vi "Create Controls within Form.vi"() -> ()   [LabVIEW 2012, in "Form.lvlib"]
uses:
  Form.lvlib
  System.Windows.Forms
panel:
  in  "停止":bool
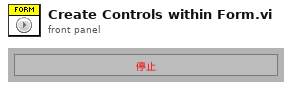
[diagram p1: front panel]
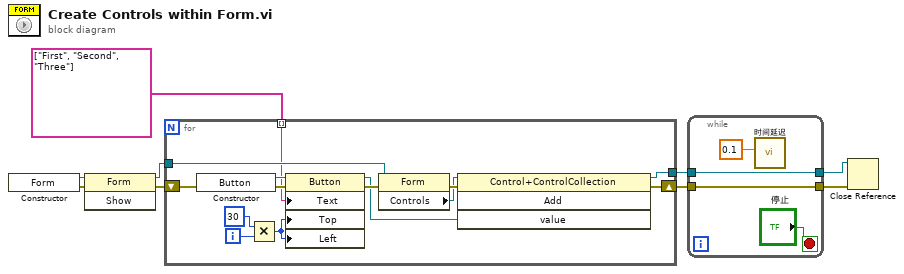
[diagram p0: block diagram]
diagram:
  n1 = constructor class="Form"() -> (reference out=w7:refnum<k24>, error out=w6:errorcluster)  [unwired: 3 in, 1 out]
  n2 = invoke class="Form" method="Show"(reference=w7, error in=w6) -> (reference out=w5:refnum<k24>, error out=w4:errorcluster)  [unwired: 1 in, 1 out]
  n3 = for {
    tunnel: w5 -> [w19]
    shift-right: [w14] -> w1
    shift-left: w4 -> [w21]
    tunnel: [w15] -> w3
    tunnel: string[] ["First", "Second", "Three"] -> [w13] mode=indexing
    i -> [w12]
    n4 = constructor class="Button"(error in=w21) -> (reference out=w23:refnum<k24>, error out=w22:errorcluster)  [unwired: 2 in, 1 out]
    n5 = Multiply(x=30, y=w12) -> (x*y=w10:i32)
    n6 = property class="Button"(reference=w23, error in=w22, "Text"=w13, "Top"=w10, "Left"=w10) -> (reference out=w16:refnum<k24>, error out=w20:errorcluster)
    n7 = property class="Form"(reference=w19, error in=w20) -> (error out=w18:errorcluster, "Controls"=w17:refnum<k24>)  [unwired: 1 out]
    n8 = invoke class="Control+ControlCollection" method="Add"(reference=w17, error in=w18, "value"=w16) -> (reference out=w15:refnum<k24>, error out=w14:errorcluster)  [unwired: 1 in, 2 out]
  }
  n9 = while {
    tunnel: w3 -> [w25]
    tunnel: w1 -> [w24]
    tunnel: [w25] -> w8
    tunnel: [w24] -> w9
    stop <- "停止" stop-if-true
    n10 = call "时间延迟"("Delay Time (s)"=0.1) -> ()  [unwired: 10 in, 1 out]
  }
  n11 = Close Reference(reference=w8, error in (no error)=w9) -> ()  [unwired: 1 out]
